vi "dht_data_receive.vi"() -> ()   [LabVIEW 2020]
uses:
  <vilib>/Instr/_visa.llb/VISA Configure Serial Port (Instr).vi
panel:
  out "read buffer":string
  out "Humidity":dbl(slide) scale=0.0..100.0
  out "Temp":dbl(slide) scale=0.0..100.0
  out "temp":dbl
  out "humid":dbl
  out "error out":errorcluster
  out "return count":u32
  in  "VISA resource name":refnum<visa-resource-name>
  in  "stop":bool
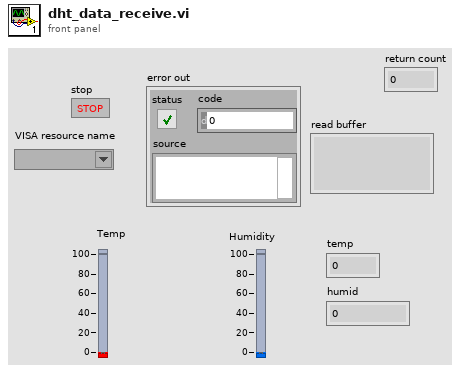
[diagram p1: front panel]
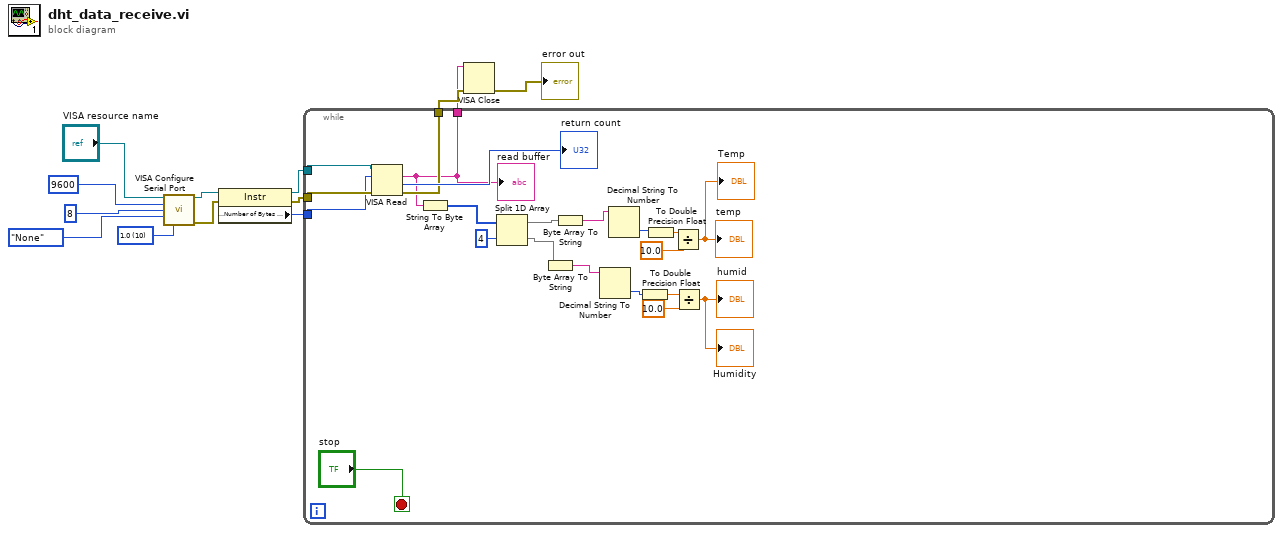
[diagram p0: block diagram]
diagram:
  w9 = u16 10 items=["1.0"=10, "1.5"=15, "2.0"=20] ("stop bits (10: 1 bit)")
  n1 = call-poly "VISA Configure Serial Port"("VISA resource name"="VISA resource name", "baud rate (9600)"=u32 9600, "data bits (8)"=u16 8, "parity (0:none)"=enum16{"None", "Odd", "Even", "Mark", "Space"}."None", "stop bits (10: 1 bit)"=w9) -> ("VISA resource name out"=w8:refnum<visa-resource-name>, "error out"=w7:errorcluster)  [unwired: 9 in]
  n2 = property class="Instr"(reference=w8, error in=w7) -> (reference out=w6:refnum<visa-resource-name>, error out=w5:errorcluster, "Serial Settings:Number of Bytes at Serial Port"=w4:u32)
  n3 = while {
    tunnel: w6 -> [w33]
    tunnel: w5 -> [w32]
    tunnel: w4 -> [w31]
    tunnel: [w14] -> w1
    tunnel: [w29] -> w3
    stop <- "stop" stop-if-true
    n4 = VISA Read(VISA resource name=w33, byte count=w31, error in (no error)=w32) -> (read buffer=w14:string, return count=→"return count":u32, error out=w29:errorcluster)  [unwired: 1 out]
    "read buffer" <- w14
    n5 = String To Byte Array(string=w14) -> (unsigned byte array=w28:u8[])
    n6 = Split 1D Array(array=w28, index=4) -> (first subarray=w26:u8[], second subarray=w24:u8[])
    n7 = Byte Array To String(unsigned byte array=w24) -> (string=w25:string)
    n8 = Byte Array To String(unsigned byte array=w26) -> (string=w23:string)
    n9 = Decimal String To Number(string=w25) -> (number=w21:i32)  [unwired: 2 in, 1 out]
    n10 = Decimal String To Number(string=w23) -> (number=w22:i32)  [unwired: 2 in, 1 out]
    n11 = To Double Precision Float(number=w21) -> (double precision float=w18:dbl)
    n12 = To Double Precision Float(number=w22) -> (double precision float=w20:dbl)
    n13 = Divide(x=w20, y=10.0) -> (x/y=→"temp" →"Temp":dbl)
    n14 = Divide(x=w18, y=10.0) -> (x/y=→"humid" →"Humidity":dbl)
  }
  n15 = VISA Close(VISA resource name=w1, error in (no error)=w3) -> (error out=→"error out":errorcluster)
